vi "Test Reset.vi"(8 "error in (no error)":errorcluster, 11 "Test Case In":refnum<class "Result Table Test.lvclass">) -> (0 "error out":errorcluster, 3 "Test Case Out":refnum<class "Result Table Test.lvclass">)   [LabVIEW 2020, in "LUnit Tests.lvlib" / "Result Table Test.lvclass"]
uses:
  Result Table Test.lvclass
  C:/Program Files (x86)/National Instruments/LabVIEW 2020/vi.lib/Astemes/LUnit/Test Case.lvclass
  source/Framework/Helper Classes/Result Table/Result Table/Result Table.lvclass
  source/Framework/Result Types/Assertion Result/Public/TypeDefs/Status.ctl
  source/Framework/Helper Classes/Result Table/Result Table/Result Table.lvclass/Result Table.ctl
  <vilib>/Astemes/LUnit/Test Case.lvclass/Test Case.ctl
  01074fa8-ee8a-411d-bc8b-fc92c4f90959.vi
  <vilib>/Astemes/LUnit/Palette/Pass.vi
  <vilib>/Astemes/LUnit/Palette/Fail.vi
  <vilib>/Astemes/LUnit/Compare Variants.vi
  <vilib>/Astemes/LUnit/Describe Comparison.vi
  <vilib>/Astemes/LUnit/Set Assertion Type.vi
  <vilib>/Astemes/LUnit/Add test result.vi
  <vilib>/Astemes/LUnit/Variant to string.vi
  <vilib>/Astemes/LUnit/LUnit Record Assertion Result.vi
  <vilib>/Astemes/LUnit/LUnit Aggregate Assertion Results.vi
  <vilib>/Astemes/LUnit/Method Result/LUnit Merge Status.vi
  <vilib>/Astemes/LUnit/LUnit Concatenate result strings.vi
  <vilib>/Utility/Data Type/Get Type Information.vi
  <vilib>/Utility/LVClass/Get LV Class Name.vi
  Result Table Test.lvclass/Result Table Test.ctl
  source/Framework/Result Types/Assertion Result/Assertion Result.lvlib
panel:
  out "Result Texts":string[](array[string])
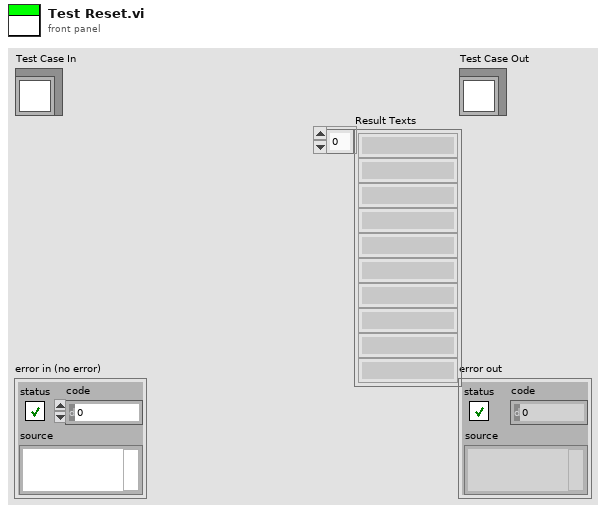
[diagram p1: front panel]
types:
  T1 = typedef "Assertion Result.lvlib/Status.ctl" = enum16{"Pass", "Fail", "Error", "Skipped", "Setup Error", "Broken", "Teardown Error"}
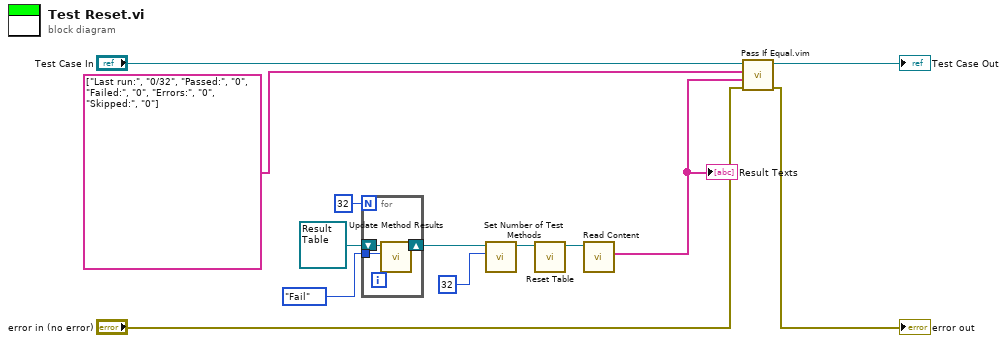
[diagram p0: block diagram]
diagram:
  n1 = for {
    N: 32 -> [_]
    tunnel: Status."Fail" ("Method Result") -> [w14]
    shift-right: [w15] -> w6
    shift-left: refnum<class "Result Table.lvclass"> refnum ("Result Table.lvclass") -> [w16]
    n2 = call "Update Method Results.vi"("Method Result"=w14, "Result Table in"=w16) -> ("Result Table out"=w15:refnum<class "Result Table.lvclass">)  [unwired: 8 in, 1 out]
  }
  n3 = call "Set Number of Test Methods.vi"("Method Count"=u32 32, "Result Table.lvclass"=w6) -> ("Result Table"=w4:refnum<class "Result Table.lvclass">)  [unwired: 8 in, 1 out]
  n4 = call "Reset Table.vi"("Result Table.lvclass"=w4) -> ("Result Table"=w1:refnum<class "Result Table.lvclass">)  [unwired: 9 in, 1 out]
  n5 = call "Read Content.vi"("Result Table in"=w1) -> ("Result Texts"=w9:string[])  [unwired: 8 in, 2 out]
  "Result Texts" <- w9
  n6 = call "Pass If Equal.vim"("error in (no error)"="error in (no error)", "Actual"=w9, "Expected"=string[] ["Last run:", "0/32", "Passed:", "0", "Failed:", "0", "Errors:", "0", "Skipped:", "0"], "LUnit Test Case In"="Test Case In") -> ("error out"=→"error out":errorcluster, "LUnit Test Case Out"=→"Test Case Out":refnum<class "Result Table Test.lvclass">)  [unwired: 6 in]
